vi "Dialog GraphSetting (Wave2).vi"(11 "波形グラフ(Wave)ref(in)":refnum<vi>) -> ()   [LabVIEW 2014]
uses:
  TypeDef/GraphSetting Appearance.ctl
  TypeDef/GraphSetting Plot.ctl
  SupportVIs/GraphSetting Scale.ctl
  TypeDef/GraphSetting DisplayFormatType.ctl
  TypeDef/GraphSetting All.ctl
  TypeDef/GraphSetting Command.ctl
  Lib/Event/Write User Event (Array).vi
  <vilib>/Utility/xml.llb/Write to XML File(string).vi
  <vilib>/Utility/xml.llb/Read From XML File(string).vi
  <vilib>/measure/NI_MABase.lvlib
panel:
  out "波形グラフ":waveform(dbl)[](graph)
  in  "ファイル読込":bool
  in  "ファイル保存":bool
  in  "タブ制御器":enum32{"外観", "スケール", "プロット"}(tab)
  in  "外観":T1
  in  "Yスケール選択":u16(ring) items=["No.", "M1回転rpm", "M2回転rpm", "M3回転rpm", "M1トルクN･m", "M2トルクN･m", "M3トルクN･m", ""]
  in  "スケール(Y軸)":T2
  in  "スケール(X軸)":T2
  in  "Xスケール選択":u16(ring) items=["時間(sec)"]
  in  "プロット":T4 {"Yスケール" items=["No.", "M1回転rpm", "M2回転rpm", "M3回転rpm", "M1トルクN･m", "M2トルクN･m", "M3トルクN･m", ""]; "Xスケール" items=["時間(sec)"]; "プロット補間" max=5 step=1; "ポイントスタイル" max=16 step=1; "太さ" max=5 step=1; "ラインスタイル" max=4 step=1}
  in  "プロット選択":u16(ring) items=["No.", "M1回転rpm", "M2回転rpm", "M3回転rpm", "M1トルクN･m", "M2トルクN･m", "M3トルクN･m", "", "", "", "", "", "", "", "", "", "", "供試体温度1℃", "供試体温度2℃", "供試体温度3℃", "動力盤温度℃", "軸受温度1℃", "軸受温度2℃", "軸受温度3℃", "", "効率"]
  in  "停止ボタン":bool
  # "スケールのスタイルとカラー"
  # "スケール係数"
  # "スケールのスタイルとカラー"
  # "スケールのスタイルとカラー"
  # "スケール係数"
  # "スケールのスタイルとカラー"
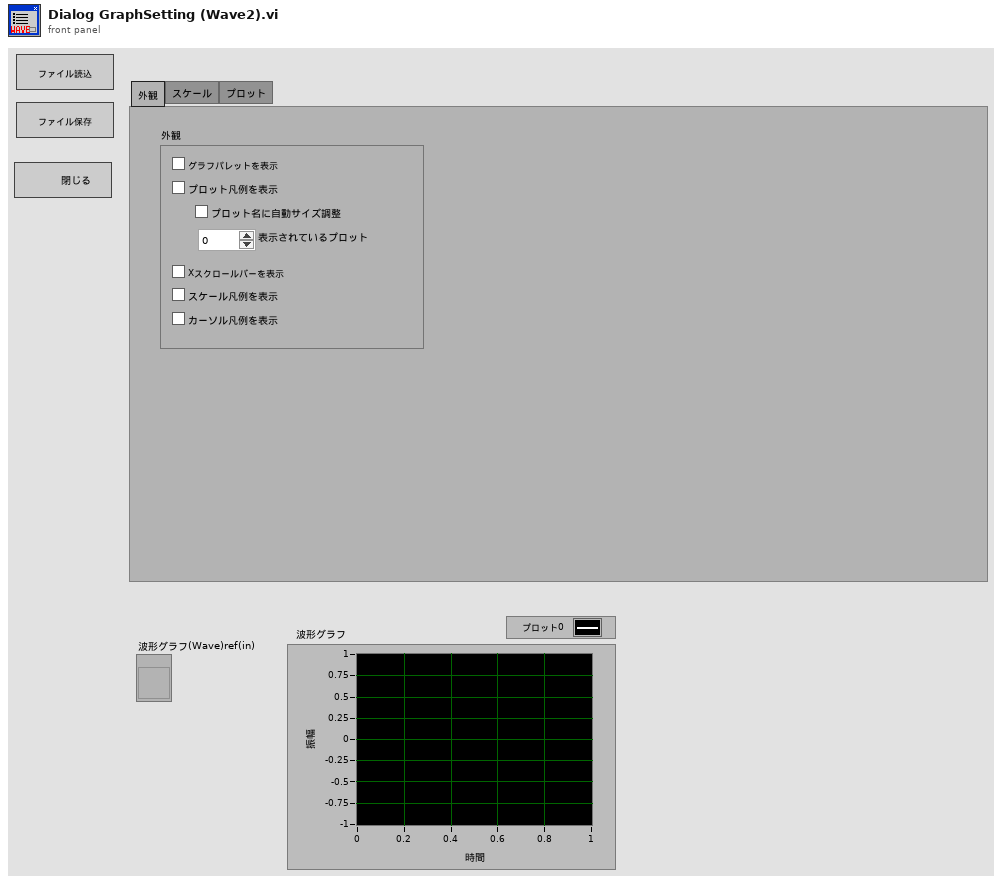
[diagram p1: front panel]
types:
  T1 = typedef "GraphSetting Appearance.ctl" = cluster{"グラフパレットを表示":bool, "プロット凡例を表示":bool, "プロット名に自動サイズ調整":bool, "表示されているプロット":u32, "Xスクロールバーを表示":bool, "スケール凡例を表示":bool, "カーソル凡例を表示":bool}
  T2 = typedef "GraphSetting Scale.ctl" = cluster{"名前":string, "スケールラベルを表示":bool, "スケールを表示":bool, "ログ":bool, "反転":bool, "自動スケール":bool, "最小":dbl, "最大":dbl, "オフセット":dbl, "乗数":dbl, "主目盛り":u32, "補助目盛り":u32, "マーカテキスト":u32, "主グリッド":u32, "補助グリッド":u32, "タイプ":T3, "小数点以下桁数":u8}
  T3 = typedef "GraphSetting DisplayFormatType.ctl" = enum8{"浮動小数点", "科学", "工学", "バイナリ", "８進数", "１６進数", "相対時間", "時間と日時", "SI"}
  T4 = typedef "GraphSetting Plot.ctl" = cluster{"名前":string, "表示":bool, "ラインスタイル":u8, "太さ":u8, "ポイントスタイル":u8, "プロット補間":u8, "ラインカラー":u32, "ポイント/塗りつぶし":u32, "Xスケール":u16, "Yスケール":u16}
  T5 = typedef "GraphSetting All.ctl" = cluster{"外観":T1, "スケールX[]":T2[], "スケールY[]":T2[], "プロット[]":T4[]}
  T6 = typedef "GraphSetting Command.ctl" = enum16{"Get(ref->ctl)", "Set(ctl->ref)"}
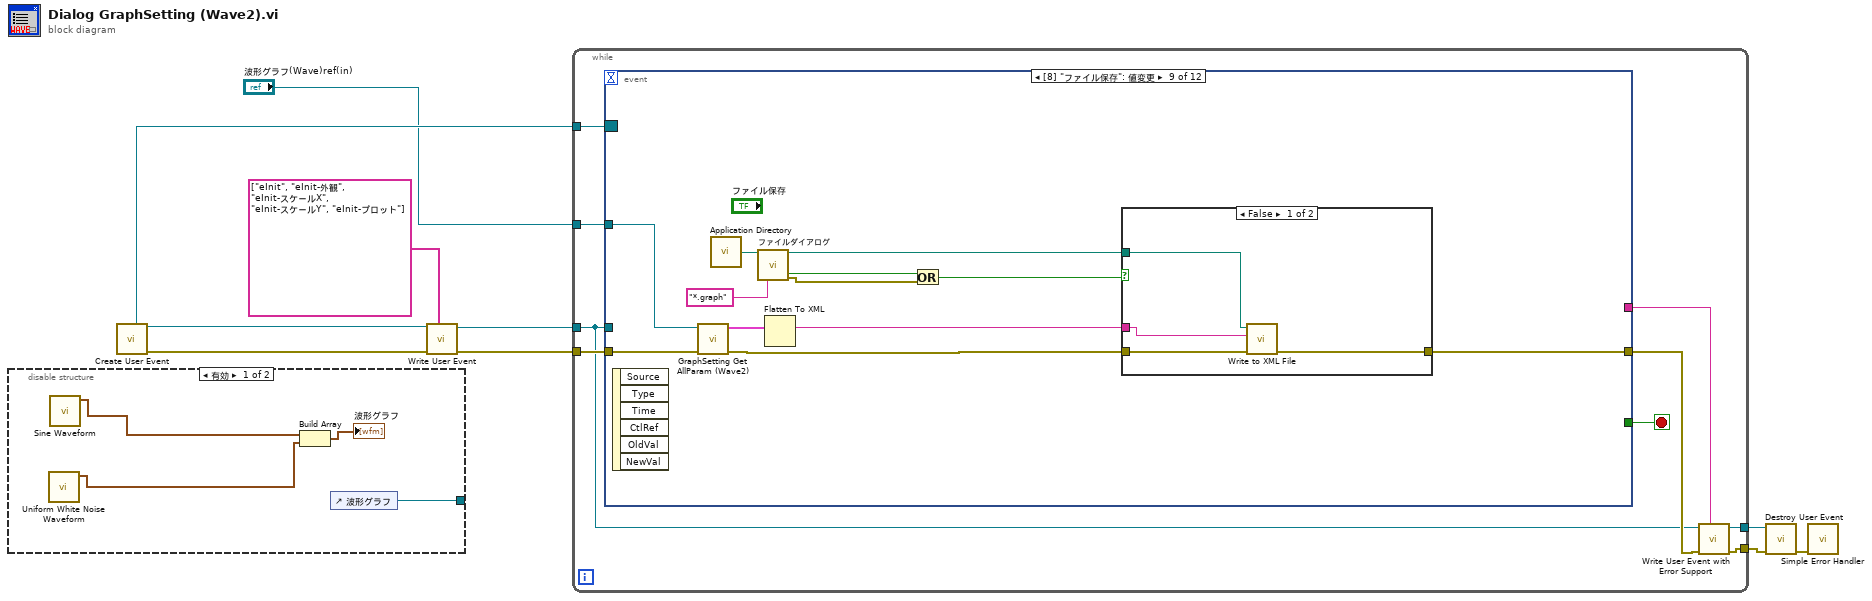
[diagram p0: block diagram]
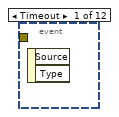
[diagram p3: hidden frame]
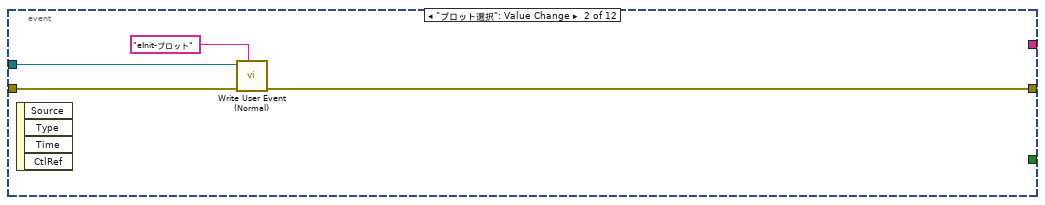
[diagram p4: hidden frame]
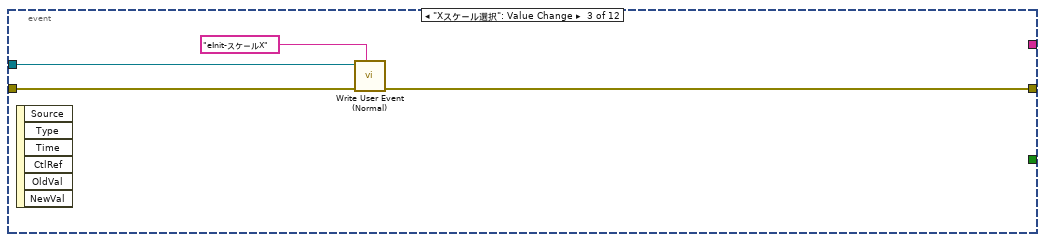
[diagram p5: hidden frame]
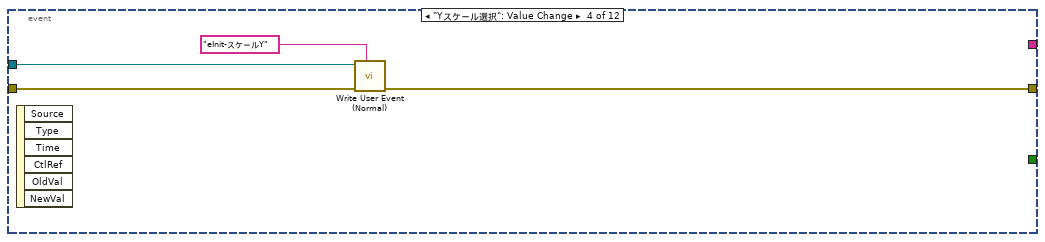
[diagram p6: hidden frame]
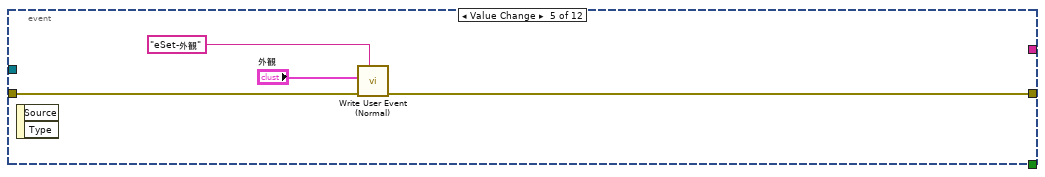
[diagram p7: hidden frame]
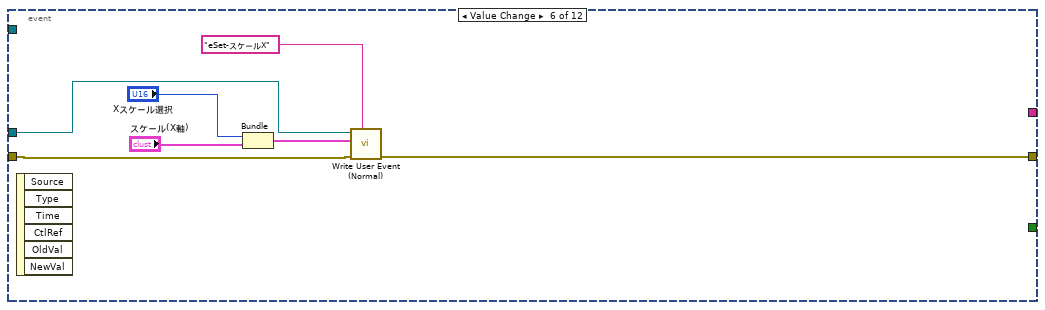
[diagram p8: hidden frame]
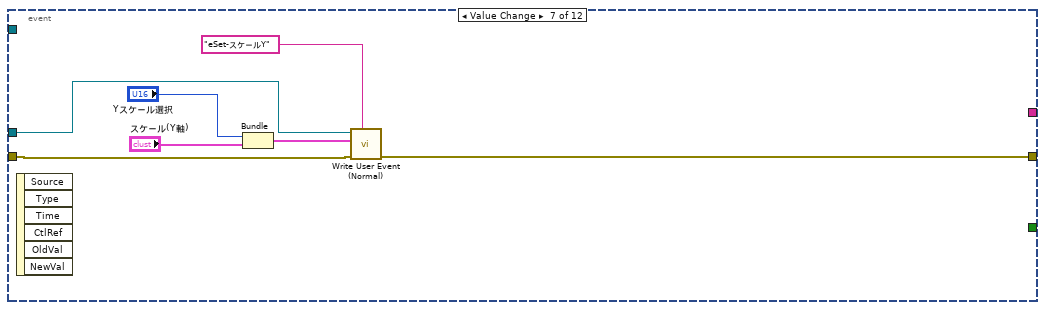
[diagram p9: hidden frame]
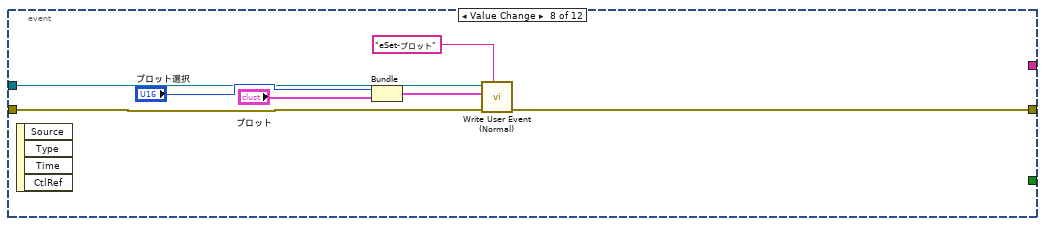
[diagram p10: hidden frame]
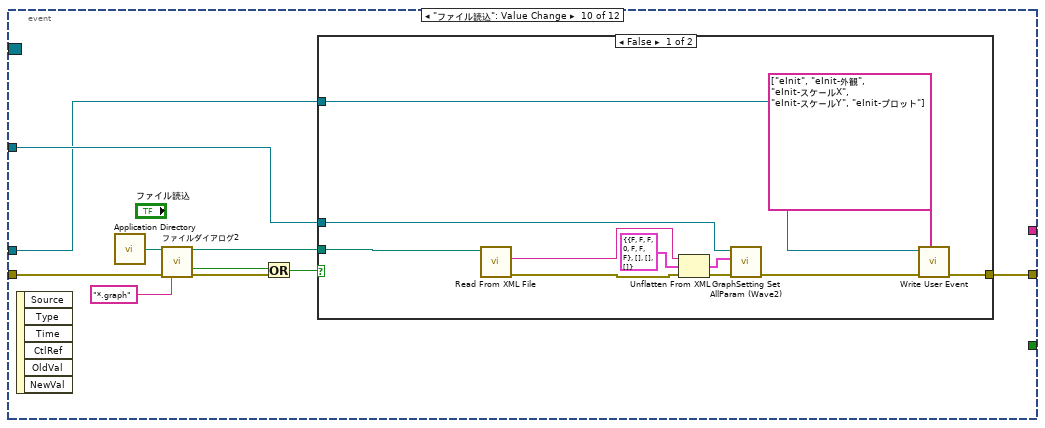
[diagram p12: hidden frame]
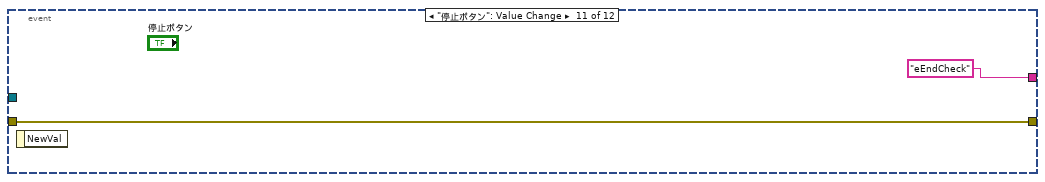
[diagram p14: hidden frame]
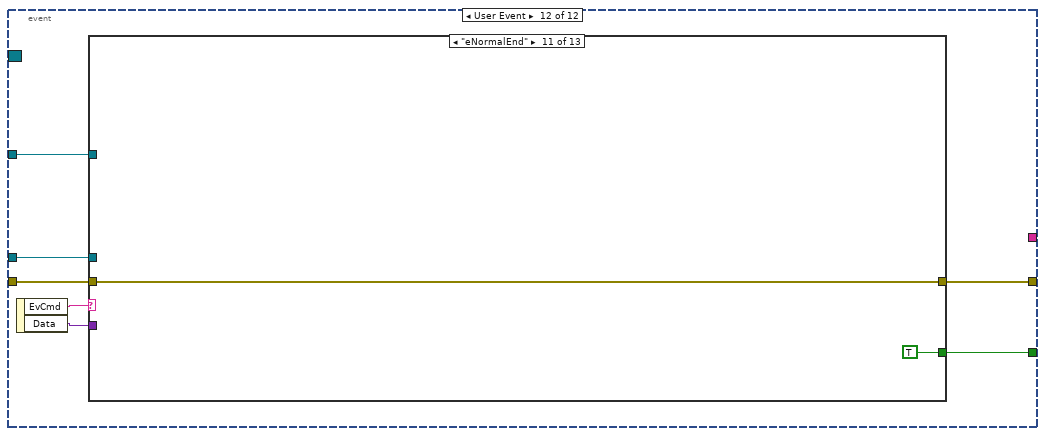
[diagram p15: hidden frame]
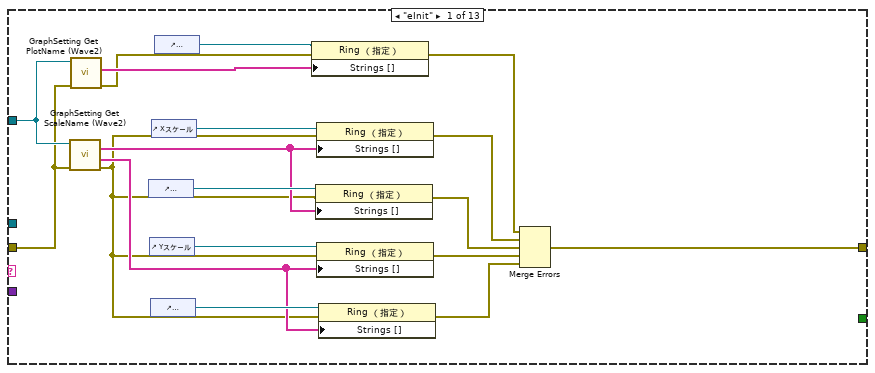
[diagram p16: hidden frame]
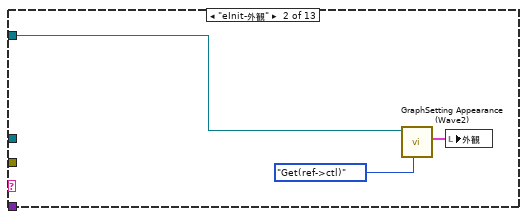
[diagram p17: hidden frame]
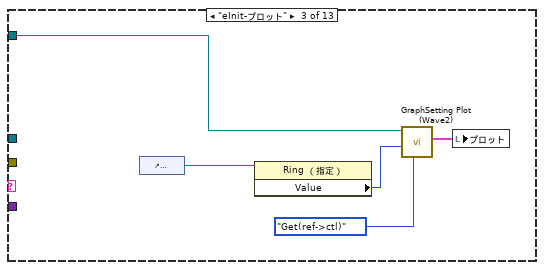
[diagram p18: hidden frame]
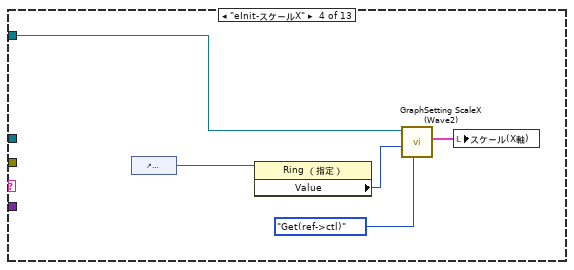
[diagram p19: hidden frame]
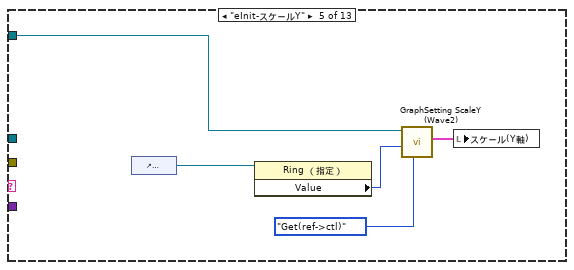
[diagram p20: hidden frame]
diagram:
  n1 = disable-structure shown="有効" {
    disable-tunnel: [w13 _] -> _
    frame Enabled {
      n2 = call <vilib>:"Uniform White Noise Waveform.vi"() -> ("signal out"=w11:waveform(dbl))  [unwired: 10 in, 1 out]
      n3 = call <vilib>:"Sine Waveform.vi"() -> ("signal out"=w12:waveform(dbl))  [unwired: 10 in, 1 out]
      n4 = Build Array(w12, w11) -> (→"波形グラフ":waveform(dbl)[])
      n5 = control-ref of="波形グラフ"() -> (w13:refnum<vi>)
    }
    frame Disabled {
    }
  }
  n6 = call "Create User Event.vi"() -> ("error out"=w8:errorcluster, "User Event"=w9:refnum<user-event>, "Event Registration Refnum"=w10:refnum<event-registration>)  [unwired: 9 in]
  n7 = call-poly "Write User Event.vi"("EvCmd[]"=string[] ["eInit", "eInit-外観", "eInit-スケールX", "eInit-スケールY", "eInit-プロット"], "エラー入力（エラーなし）"=w8, "ユーザイベント入力"=w9) -> ("エラー出力"=w4:errorcluster, "ユーザイベント出力"=w5:refnum<user-event>)  [unwired: 7 in]
  n8 = while {
    tunnel: w4 -> [w22]
    tunnel: w10 -> [w23]
    tunnel: [w19] -> w7
    tunnel: w5 -> [w15]
    tunnel: "波形グラフ(Wave)ref(in)" -> [w21]
    tunnel: [w16] -> w2
    stop <- w17 stop-if-true
    n9 = event shown="[8] \"ファイル保存\": 値変更" {
      selector: w23 -> [_ _ _ _ _ _ _ _ _ _ _ _]
      dyn-events: _ -> [_ _ _ _ _ _ _ _ _ _ _ _]
      timeout: _ -> [_ _ _ _ _ _ _ _ _ _ _ _]
      tunnel: [_ _ _ _ _ _ _ _ _ _ _ w103] -> w17
      tunnel: [_ w25 w29 w32 w36 w41 w48 w55 w68 w82 w99 w104] -> w20
      tunnel: w22 -> [_ w26 w31 w34 w37 w40 w49 w56 w65 w85 w99 w105]
      tunnel: w15 -> [_ w27 w30 w33 _ w44 w50 w57 _ w81 _ w102]
      tunnel: w21 -> [_ _ _ _ _ _ _ _ w64 w83 _ w101]
      tunnel: [_ _ _ _ _ _ _ _ _ _ "eEndCheck" ("EvCmd") _] -> w18
      event Timeout {
        n10 = event-data() -> ()  [unwired: 1 in, 2 out]
      }
      event "プロット選択": Value Change {
        n11 = event-data() -> ()  [unwired: 1 in, 4 out]
        n12 = call "Write User Event (Normal).vi"("EvCmd"="eInit-プロット", "エラー入力（エラーなし）"=w26, "ユーザイベント入力"=w27) -> ("エラー出力"=w25:errorcluster)  [unwired: 7 in, 1 out]
      }
      event "Xスケール選択": Value Change {
        n13 = event-data() -> ()  [unwired: 1 in, 6 out]
        n14 = call "Write User Event (Normal).vi"("EvCmd"="eInit-スケールX", "エラー入力（エラーなし）"=w31, "ユーザイベント入力"=w30) -> ("エラー出力"=w29:errorcluster)  [unwired: 7 in, 1 out]
      }
      event "Yスケール選択": Value Change {
        n15 = event-data() -> ()  [unwired: 1 in, 6 out]
        n16 = call "Write User Event (Normal).vi"("EvCmd"="eInit-スケールY", "エラー入力（エラーなし）"=w34, "ユーザイベント入力"=w33) -> ("エラー出力"=w32:errorcluster)  [unwired: 7 in, 1 out]
      }
      event Value Change {
        n17 = event-data() -> ()  [unwired: 1 in, 2 out]
        n18 = call "Write User Event (Normal).vi"("EvCmd"="eSet-外観", "エラー入力（エラーなし）"=w37, "データ"="外観") -> ("エラー出力"=w36:errorcluster)  [unwired: 7 in, 1 out]
      }
      event Value Change {
        n19 = event-data() -> ()  [unwired: 1 in, 6 out]
        n20 = Bundle("Xスケール選択"="Xスケール選択", "スケール(X軸)"="スケール(X軸)") -> (w45:cluster{"Xスケール選択":u16, "スケール(X軸)":T2})  [unwired: 1 in]
        n21 = call "Write User Event (Normal).vi"("EvCmd"="eSet-スケールX", "エラー入力（エラーなし）"=w40, "データ"=w45, "ユーザイベント入力"=w44) -> ("エラー出力"=w41:errorcluster)  [unwired: 6 in, 1 out]
      }
      event Value Change {
        n22 = event-data() -> ()  [unwired: 1 in, 6 out]
        n23 = Bundle("Yスケール選択"="Yスケール選択", "スケール(Y軸)"="スケール(Y軸)") -> (w51:cluster{"Yスケール選択":u16, "スケール(Y軸)":T2})  [unwired: 1 in]
        n24 = call "Write User Event (Normal).vi"("EvCmd"="eSet-スケールY", "エラー入力（エラーなし）"=w49, "データ"=w51, "ユーザイベント入力"=w50) -> ("エラー出力"=w48:errorcluster)  [unwired: 6 in, 1 out]
      }
      event Value Change {
        n25 = event-data() -> ()  [unwired: 1 in, 4 out]
        n26 = Bundle("プロット選択"="プロット選択", "プロット"="プロット") -> (w58:cluster{"プロット選択":u16, "プロット":T4})  [unwired: 1 in]
        n27 = call "Write User Event (Normal).vi"("EvCmd"="eSet-プロット", "エラー入力（エラーなし）"=w56, "データ"=w58, "ユーザイベント入力"=w57) -> ("エラー出力"=w55:errorcluster)  [unwired: 6 in, 1 out]
      }
      event "ファイル保存": Value Change {
        n28 = event-data() -> ()  [unwired: 1 in, 6 out]
        n29 = call "GraphSetting Get AllParam (Wave2).vi"("エラー入力（エラーなし）"=w65, "波形グラフ(Wave)ref(in)"=w64) -> ("エラー出力"=w67:errorcluster, "クラスタ"=w66:cluster{"外観(out)":T1, T2[], T2[], T4[]})  [unwired: 8 in]
        n30 = call <vilib>:"Application Directory.vi"() -> ("Application Directory"=w71:path)
        n31 = call "ファイルダイアログ"("start path"=w71, "pattern (all files)"="*.graph") -> ("selected path"=w69:path, "cancelled"=w63:bool, "error out"=w62:errorcluster)  [unwired: 10 in, 1 out]
        n32 = Flatten To XML(anything=w66) -> (xml string=w70:string)
        n33 = Or(x=w63, y=w62) -> (x .or. y?=w61:bool)
        n34 = case shown="FALSE" w61 {
          tunnel: w69 -> [w76 _]
          tunnel: w70 -> [w75 _]
          tunnel: w67 -> [w73 w77]
          tunnel: [w74 w77] -> w68
          frame False {
            n35 = call-poly <vilib>:"Write to XML File.vi"("error in (no error)"=w73, "XML Input"=w75, "XML File Path"=w76) -> ("error out"=w74:errorcluster)  [unwired: 6 in, 2 out]
          }
          frame True {
          }
        }
      }
      event "ファイル読込": Value Change {
        n36 = event-data() -> ()  [unwired: 1 in, 6 out]
        n37 = call <vilib>:"Application Directory.vi"() -> ("Application Directory"=w87:path)
        n38 = call "ファイルダイアログ2"("start path"=w87, "error in"=w85, "pattern (all files)"="*.graph") -> ("selected path"=w84:path, "cancelled"=w79:bool, "error out"=w80:errorcluster)  [unwired: 9 in, 1 out]
        n39 = Or(x=w79, y=w80) -> (x .or. y?=w78:bool)
        n40 = case shown="FALSE" w78 {
          tunnel: w84 -> [w96 _]
          tunnel: w83 -> [w92 _]
          tunnel: [w89 _] -> w82
          tunnel: w81 -> [w91 _]
          frame False {
            n41 = call-poly <vilib>:"Read From XML File.vi"("XML File Path"=w96) -> ("error out"=w95:errorcluster, "XML Elements"=w97:string)  [unwired: 8 in, 1 out]
            n42 = Unflatten From XML(xml string=w97, type=T5 {"外観"={"グラフパレットを表示"=FALSE, "プロット凡例を表示"=FALSE, "プロット名に自動サイズ調整"=FALSE, "表示されているプロット"=0, "Xスクロールバーを表示"=FALSE, "スケール凡例を表示"=FALSE, "カーソル凡例を表示"=FALSE}, "スケールX[]"=[], "スケールY[]"=[], "プロット[]"=[]} ("出力クラスタ"), error in (no error)=w95) -> (value=w94:T5, error out=w93:errorcluster)
            n43 = call "GraphSetting Set AllParam (Wave2).vi"("error in (no error)"=w93, "Chartグラフパラメータ"=w94, "波形グラフ(Wave)ref(in)"=w92) -> ("error out"=w90:errorcluster)  [unwired: 8 in]
            n44 = call-poly "Write User Event.vi"("EvCmd[]"=string[] ["eInit", "eInit-外観", "eInit-スケールX", "eInit-スケールY", "eInit-プロット"], "エラー入力（エラーなし）"=w90, "ユーザイベント入力"=w91) -> ("エラー出力"=w89:errorcluster)  [unwired: 7 in, 1 out]
          }
          frame True {
          }
        }
      }
      event "停止ボタン": Value Change {
        n45 = event-data() -> ()  [unwired: 1 in, 1 out]
      }
      event User Event {
        n46 = event-data() -> ("EvCmd"=w107:string, "Data"=w106:variant)  [unwired: 1 in]
        n47 = case shown="\"eNormalEnd\"" w107 {
          selector: w107 -> [_ _ _ _ _ _ _ _ _ _ _ _ w191]
          tunnel: w106 -> [_ _ _ _ _ w148 w156 w167 w177 _ _ w190 _]
          tunnel: w105 -> [w117 _ _ _ _ w146 w158 w166 w176 w181 w185 w188 _]
          tunnel: [w108 _ _ _ _ w144 w151 w160 w170 w180 w185 _ _] -> w104
          tunnel: [_ _ _ _ _ _ _ _ _ _ TRUE TRUE _] -> w103
          tunnel: w102 -> [_ _ _ _ _ _ _ _ _ w183 _ _ _]
          tunnel: w101 -> [w120 w128 w133 w138 w143 w149 w152 w164 w174 _ _ _ _]
          frame "eInit" {
            n48 = call "GraphSetting Get ScaleName (Wave2).vi"("error in (no error)"=w117, "波形グラフ(Wave)ref(in)"=w120) -> ("error out"=w114:errorcluster, "Y軸名称[]"=w116:string[], "X軸名称[]"=w123:string[])  [unwired: 7 in]
            n49 = call "GraphSetting Get PlotName (Wave2).vi"("error in (no error)"=w117, "波形グラフ(Wave)ref(in)"=w120) -> ("error out"=w115:errorcluster, "プロット名称[]"=w118:string[])  [unwired: 8 in]
            n50 = control-ref of="Xスケール選択"() -> (w124:refnum<vi>)
            n51 = control-ref of="Yスケール"() -> (w121:refnum<vi>)
            n52 = control-ref of="Yスケール選択"() -> (w122:refnum<vi>)
            n53 = control-ref of="Xスケール"() -> (w125:refnum<vi>)
            n54 = control-ref of="プロット選択"() -> (w119:refnum<vi>)
            n55 = property class="Ring （指定）"(reference=w119, error in=w115, "Strings []"=w118) -> (error out=w113:errorcluster)  [unwired: 1 out]
            n56 = property class="Ring （指定）"(reference=w124, error in=w114, "Strings []"=w123) -> (error out=w111:errorcluster)  [unwired: 1 out]
            n57 = property class="Ring （指定）"(reference=w125, error in=w114, "Strings []"=w123) -> (error out=w112:errorcluster)  [unwired: 1 out]
            n58 = property class="Ring （指定）"(reference=w121, error in=w114, "Strings []"=w116) -> (error out=w110:errorcluster)  [unwired: 1 out]
            n59 = property class="Ring （指定）"(reference=w122, error in=w114, "Strings []"=w116) -> (error out=w109:errorcluster)  [unwired: 1 out]
            n60 = Merge Errors(w113, w112, w111, w110, w109) -> (w108:errorcluster)
          }
          frame "eInit-外観" {
            n61 = call "GraphSetting Appearance (Wave2).vi"("コマンド"=GraphSetting_Command."Get(ref->ctl)", "波形グラフ(Wave)ref(in)"=w128) -> ("外観(out)"=w127:T1)  [unwired: 8 in, 1 out]
            n62 = local write "外観"(w127) -> ()
          }
          frame "eInit-プロット" {
            n63 = control-ref of="プロット選択"() -> (w132:refnum<vi>)
            n64 = property class="Ring （指定）"(reference=w132) -> ("Value"=w131:u16)  [unwired: 1 in, 2 out]
            n65 = call "GraphSetting Plot (Wave2).vi"("コマンド"=GraphSetting_Command."Get(ref->ctl)", "アクティブプロット"=w131, "波形グラフ(Wave)ref(in)"=w133) -> ("プロット(out)"=w129:T4)  [unwired: 7 in, 1 out]
            n66 = local write "プロット"(w129) -> ()
          }
          frame "eInit-スケールX" {
            n67 = control-ref of="Xスケール選択"() -> (w137:refnum<vi>)
            n68 = property class="Ring （指定）"(reference=w137) -> ("Value"=w136:u16)  [unwired: 1 in, 2 out]
            n69 = call "GraphSetting ScaleX (Wave2).vi"("コマンド"=GraphSetting_Command."Get(ref->ctl)", "アクティブスケール(X)"=w136, "波形グラフ(Wave)ref(in)"=w138) -> ("スケール(out)"=w134:T2)  [unwired: 7 in, 1 out]
            n70 = local write "スケール(X軸)"(w134) -> ()
          }
          frame "eInit-スケールY" {
            n71 = control-ref of="Yスケール選択"() -> (w142:refnum<vi>)
            n72 = property class="Ring （指定）"(reference=w142) -> ("Value"=w141:u16)  [unwired: 1 in, 2 out]
            n73 = call "GraphSetting ScaleY (Wave2).vi"("コマンド"=GraphSetting_Command."Get(ref->ctl)", "アクティブスケールY"=w141, "波形グラフ(Wave)ref(in)"=w143) -> ("スケール(out)"=w139:T2)  [unwired: 7 in, 1 out]
            n74 = local write "スケール(Y軸)"(w139) -> ()
          }
          frame "eSet-外観" {
            n75 = Variant To Data(error in=w146, Variant=w148) -> (data=w147:T1, error out=w145:errorcluster)  [unwired: 1 in]
            n76 = call "GraphSetting Appearance (Wave2).vi"("コマンド"=GraphSetting_Command."Set(ctl->ref)", "error in (no error)"=w145, "外観(in)"=w147, "波形グラフ(Wave)ref(in)"=w149) -> ("error out"=w144:errorcluster)  [unwired: 6 in, 1 out]
          }
          frame "eSet-スケールX" {
            n77 = Variant To Data(type=cluster{"Xスケール選択":u16, "スケール(X軸)":T2} {"Xスケール選択"=0, "スケール(X軸)"={"名前"="", "スケールラベルを表示"=FALSE, "スケールを表示"=FALSE, "ログ"=FALSE, "反転"=FALSE, "自動スケール"=FALSE, "最小"=0.0, "最大"=0.0, "オフセット"=0.0, "乗数"=0.0, "主目盛り"=0, "補助目盛り"=0, "マーカテキスト"=0, "主グリッド"=0, "補助グリッド"=0, "タイプ"=enum."浮動小数点", "小数点以下桁数"=0}} ("出力クラスタ"), Variant=w156) -> (data=w155:cluster{"Xスケール選択":u16, "スケール(X軸)":T2})  [unwired: 1 in, 1 out]
            n78 = Unbundle(w155) -> ("Xスケール選択"=w153:u16, "スケール(X軸)"=w154:T2)
            n79 = call "GraphSetting ScaleX (Wave2).vi"("コマンド"=GraphSetting_Command."Set(ctl->ref)", "error in (no error)"=w158, "アクティブスケール(X)"=w153, "スケール(in)"=w154, "波形グラフ(Wave)ref(in)"=w152) -> ("error out"=w151:errorcluster)  [unwired: 5 in, 1 out]
          }
          frame "eSet-スケールY" {
            n80 = Variant To Data(error in=w166, type=cluster{"Xスケール選択":u16, "スケール(X軸)":T2} {"Xスケール選択"=0, "スケール(X軸)"={"名前"="", "スケールラベルを表示"=FALSE, "スケールを表示"=FALSE, "ログ"=FALSE, "反転"=FALSE, "自動スケール"=FALSE, "最小"=0.0, "最大"=0.0, "オフセット"=0.0, "乗数"=0.0, "主目盛り"=0, "補助目盛り"=0, "マーカテキスト"=0, "主グリッド"=0, "補助グリッド"=0, "タイプ"=enum."浮動小数点", "小数点以下桁数"=0}} ("出力クラスタ"), Variant=w167) -> (data=w165:cluster{"Xスケール選択":u16, "スケール(X軸)":T2}, error out=w161:errorcluster)
            n81 = Unbundle(w165) -> ("Xスケール選択"=w162:u16, "スケール(X軸)"=w163:T2)
            n82 = call "GraphSetting ScaleY (Wave2).vi"("コマンド"=GraphSetting_Command."Set(ctl->ref)", "error in (no error)"=w161, "アクティブスケールY"=w162, "スケール(in)"=w163, "波形グラフ(Wave)ref(in)"=w164) -> ("error out"=w160:errorcluster)  [unwired: 5 in, 1 out]
          }
          frame "eSet-プロット" {
            n83 = Variant To Data(error in=w176, type=cluster{"プロット選択":u16, "プロット":T4} {"プロット選択"=0, "プロット"={"名前"="", "表示"=FALSE, "ラインスタイル"=0, "太さ"=0, "ポイントスタイル"=0, "プロット補間"=0, "ラインカラー"=0, "ポイント/塗りつぶし"=0, "Xスケール"=0, "Yスケール"=0}} ("出力クラスタ"), Variant=w177) -> (data=w175:cluster{"プロット選択":u16, "プロット":T4}, error out=w173:errorcluster)
            n84 = Unbundle(w175) -> ("プロット選択"=w172:u16, "プロット"=w171:T4)
            n85 = call "GraphSetting Plot (Wave2).vi"("コマンド"=GraphSetting_Command."Set(ctl->ref)", "error in (no error)"=w173, "アクティブプロット"=w172, "プロット(in)"=w171, "波形グラフ(Wave)ref(in)"=w174) -> ("error out"=w170:errorcluster)  [unwired: 5 in, 1 out]
          }
          frame "eEndCheck" {
            n86 = call "Write User Event (Normal).vi"("EvCmd"="eNormalEnd", "エラー入力（エラーなし）"=w181, "ユーザイベント入力"=w183) -> ("エラー出力"=w180:errorcluster)  [unwired: 7 in, 1 out]
          }
          frame "eNormalEnd" {
          }
          frame "eErrorEnd" {
            n87 = Variant To Data(error in=w188, type=errorcluster {"status"=FALSE, "code"=0, "source"=""} ("エラー定数"), Variant=w190) -> (data=w187:errorcluster)  [unwired: 1 out]
            n88 = call <vilib>:"Simple Error Handler.vi"("error in (no error)"=w187) -> ()  [unwired: 4 in, 5 out]
          }
          frame Default {
            n89 = call "DialogProgramError.vi"("エラー内容"="ユーザイベント例外" ("エラー詳細"), "エラー詳細"=w191) -> ()  [unwired: 9 in, 1 out]
          }
        }
      }
    }
    n90 = call "Write User Event with Error Support.vi"("EvCmd"=w18, "エラー入力（エラーなし）"=w20, "ユーザイベント入力"=w15) -> ("エラー出力"=w19:errorcluster, "ユーザイベント出力"=w16:refnum<user-event>)  [unwired: 7 in]
  }
  n91 = call "Destroy User Event.vi"("error in (no error)"=w7, "User Event"=w2) -> ("error out"=w6:errorcluster)  [unwired: 9 in]
  n92 = call <vilib>:"Simple Error Handler.vi"("error in (no error)"=w6) -> ()  [unwired: 4 in, 5 out]
